vi "SetScanSource.vi"(8 "Error In":errorcluster, 10 "Scan Source":T1, 11 "Keithley 7001 In":refnum<visa-resource-name>) -> (0 "Error Out":errorcluster, 3 "Keithley 7001 Out":refnum<visa-resource-name>)   [LabVIEW 2012, in "Keithley-7001.lvlib"]
uses:
  Keithley-7001.lvlib
  Controls/ScanSource.ctl
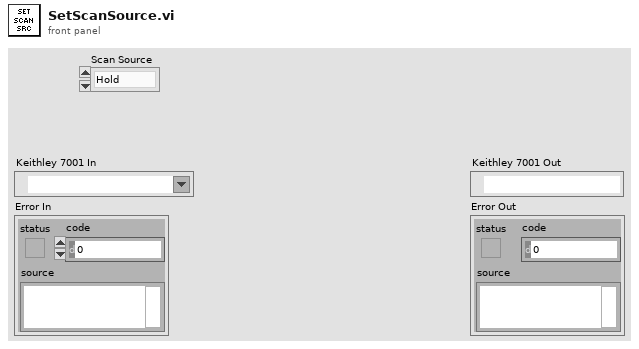
[diagram p1: front panel]
types:
  T1 = typedef "Keithley-7001.lvlib/ScanSource.ctl" = enum16{"Hold", "Immediate", "Timer", "Manual", "Bus", "TLink", "External"}
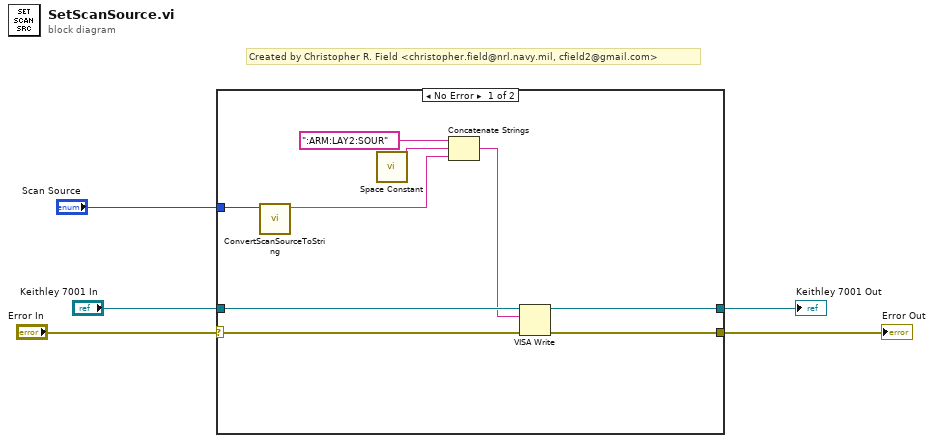
[diagram p0: block diagram]
diagram:
  # "Created by Christopher R. Field <christopher.field@nrl.navy.mil, cfield2@gmail.com>"
  n1 = case shown="No Error" "Error In" {
    selector: "Error In" -> [w8 w15]
    tunnel: "Keithley 7001 In" -> [w14 w16]
    tunnel: [w13 w16] -> w4
    tunnel: [w12 w15] -> w3
    tunnel: "Scan Source" -> [w7 _]
    frame No Error {
      n2 = call "ConvertScanSourceToString.vi"("Scan Source"=w7) -> ("String"=w6:string)  [unwired: 10 in]
      n3 = call <vilib>:"Space Constant.vi"() -> ("String"=w10:string)
      n4 = Concatenate Strings(":ARM:LAY2:SOUR" ("write buffer"), w10, w6) -> (w9:string)
      n5 = VISA Write(VISA resource name=w14, write buffer=w9, error in (no error)=w8) -> (VISA resource name out=w13:refnum<visa-resource-name>, error out=w12:errorcluster)  [unwired: 1 out]
    }
    frame Error {
    }
  }
  "Keithley 7001 Out" <- w4
  "Error Out" <- w3
